vi "LD2018_ブロック崩し_当たり判定.vi"(0 "file path (dialog if empty)":path, 5 "Ball座標":T1, 7 "ブロックReferences":refnum<vi>[][](array[refnum]), 9 "ブロック配列in":bool[][](array[boolean]), 11 "方向in":i32, 12 "行":i32=10, 13 "列":i32=10) -> (6 "Hit?":bool, 10 "ブロック配列":bool[][](array[boolean]), 15 "方向out":i32)   [LabVIEW 2016]
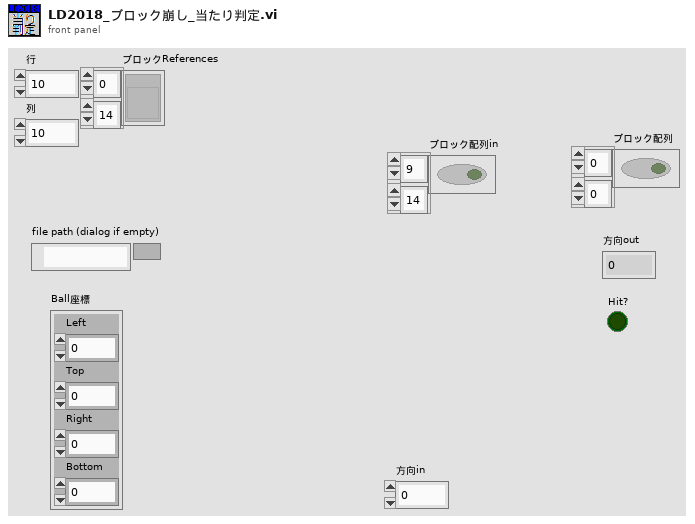
[diagram p1: front panel]
types:
  T1 = cluster{"Left":dbl, "Top":dbl, "Right":dbl, "Bottom":dbl}
  T2 = cluster{"Left":i16, "Top":i16, "Right":i16, "Bottom":i16}
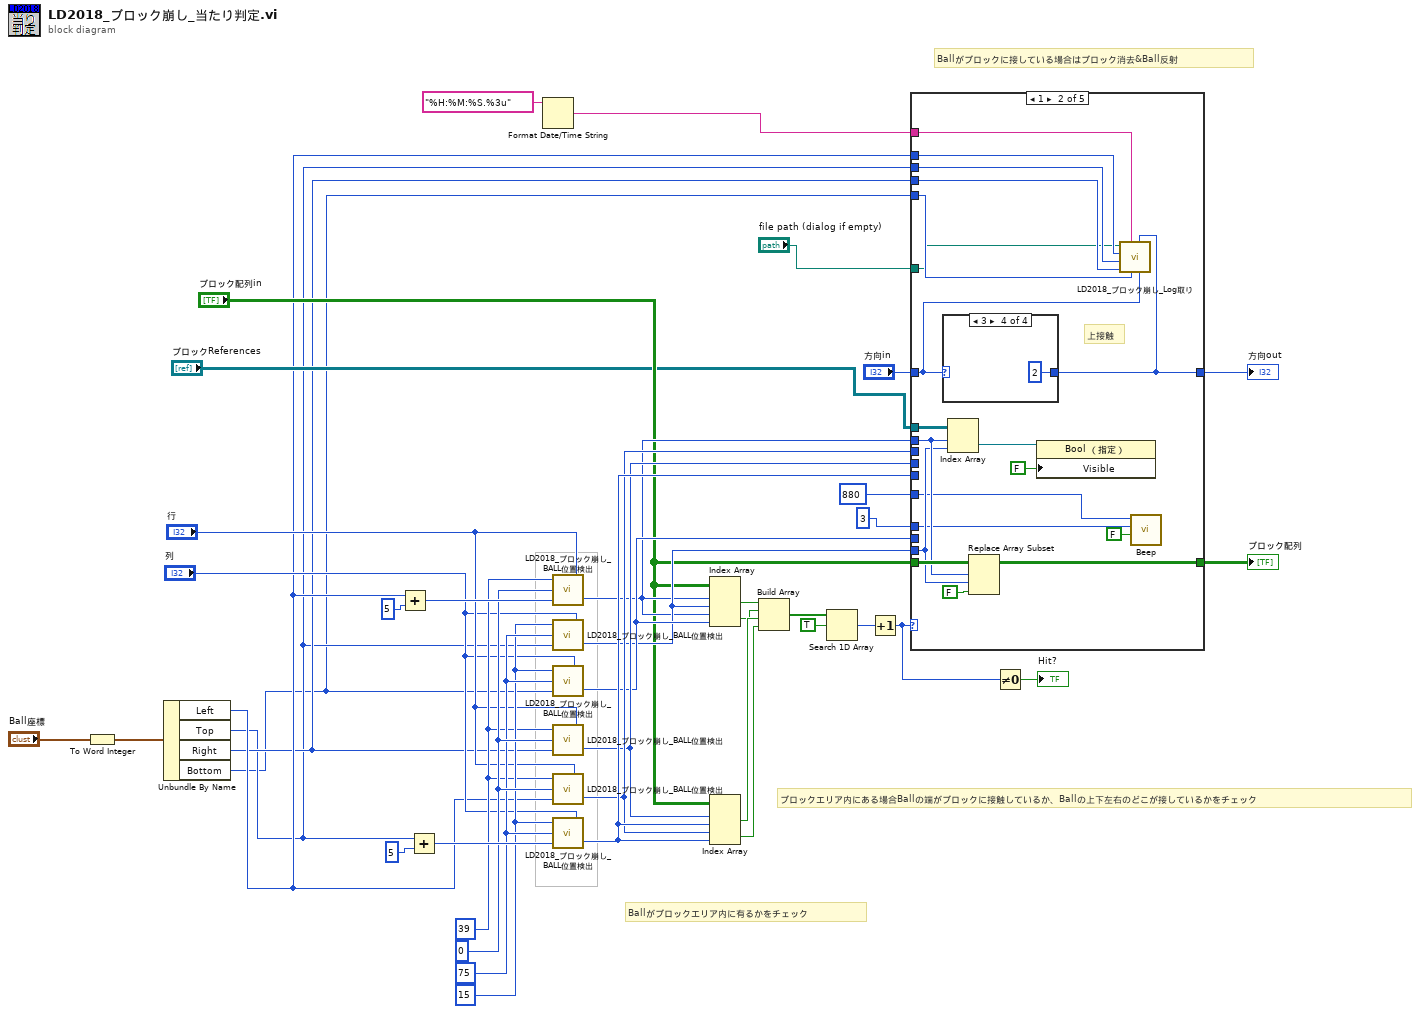
[diagram p0: block diagram]
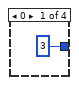
[diagram p3: hidden frame]
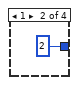
[diagram p4: hidden frame]
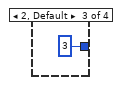
[diagram p5: hidden frame]
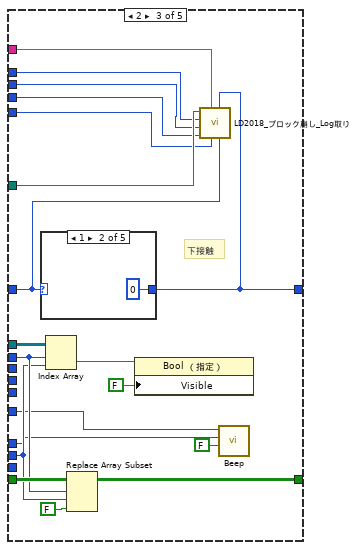
[diagram p6: hidden frame]
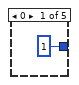
[diagram p7: hidden frame]
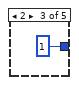
[diagram p8: hidden frame]
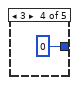
[diagram p9: hidden frame]
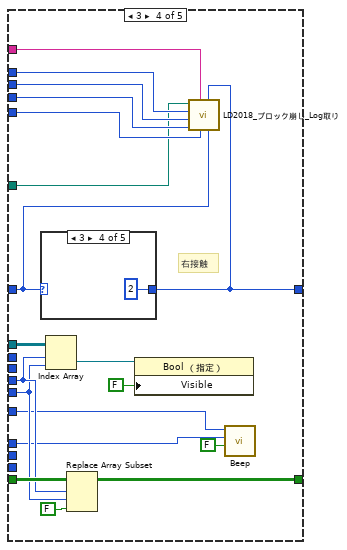
[diagram p11: hidden frame]
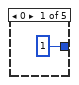
[diagram p12: hidden frame]
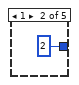
[diagram p13: hidden frame]
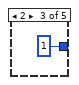
[diagram p14: hidden frame]
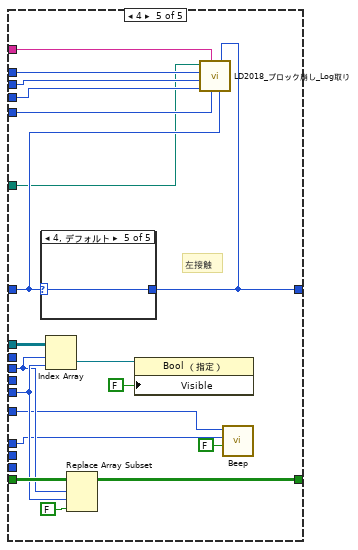
[diagram p16: hidden frame]
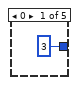
[diagram p17: hidden frame]
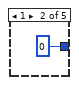
[diagram p18: hidden frame]
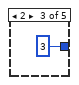
[diagram p19: hidden frame]
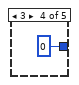
[diagram p20: hidden frame]
diagram:
  w19 = 75 ("オフセット")
  w20 = 0 ("オフセット")
  w17 = 39 ("幅/高さ")
  w18 = 15 ("幅/高さ")
  # "Ballがブロックに接している場合はブロック消去&Ball反射"
  # "ブロックエリア内にある場合Ballの端がブロックに接触しているか、Ballの上下左右のどこが接しているかをチェック"
  # "Ballがブロックエリア内に有るかをチェック"
  n1 = To Word Integer(number="Ball座標") -> (16bit integer=w3:T2)
  n2 = Unbundle By Name(w3) -> ("Left"=w7:i16, "Top"=w5:i16, "Right"=w6:i16, "Bottom"=w4:i16)
  n3 = Add(x=w7, y=i16 5) -> (x+y=w23:i16)
  n4 = Add(x=w5, y=i16 5) -> (x+y=w24:i16)
  n5 = Format Date/Time String(time format string (%c)="%H:%M:%S.%3u" ("時間形式文字列（%c）")) -> (date/time string=w11:string)  [unwired: 2 in]
  n6 = call "LD2018_ブロック崩し_BALL位置検出.vi"("行/列数"="行", "BALL座標"=w23, "オフセット"=w20, "幅/高さ"=w17) -> ("位置"=w33:i32)
  n7 = call "LD2018_ブロック崩し_BALL位置検出.vi"("行/列数"="列", "BALL座標"=w5, "オフセット"=w19, "幅/高さ"=w18) -> ("位置"=w34:i32)
  n8 = call "LD2018_ブロック崩し_BALL位置検出.vi"("行/列数"="列", "BALL座標"=w4, "オフセット"=w19, "幅/高さ"=w18) -> ("位置"=w35:i32)
  n9 = call "LD2018_ブロック崩し_BALL位置検出.vi"("行/列数"="行", "BALL座標"=w6, "オフセット"=w20, "幅/高さ"=w17) -> ("位置"=w36:i32)
  n10 = call "LD2018_ブロック崩し_BALL位置検出.vi"("行/列数"="行", "BALL座標"=w7, "オフセット"=w20, "幅/高さ"=w17) -> ("位置"=w37:i32)
  n11 = call "LD2018_ブロック崩し_BALL位置検出.vi"("行/列数"="列", "BALL座標"=w24, "オフセット"=w19, "幅/高さ"=w18) -> ("位置"=w38:i32)
  n12 = Index Array(array="ブロック配列in", index (row) #1=w33, index (col) #1=w34, index (row) #2=w33, index (col) #2=w35) -> (element #1=w26:bool, element #2=w27:bool)
  n13 = Index Array(array="ブロック配列in", index (row) #1=w36, index (col) #1=w38, index (row) #2=w37, index (col) #2=w38) -> (element #1=w28:bool, element #2=w29:bool)
  n14 = Build Array(w26, w27, w28, w29) -> (w30:bool[])
  n15 = Search 1D Array(1D array=w30, element=TRUE ("要素")) -> (index of element=w32:i32)  [unwired: 1 in]
  n16 = Increment(x=w32) -> (x+1=w10:i32)
  n17 = case shown="1" w10 {
    tunnel: w33 -> [_ w59 w82 _ _]
    tunnel: w34 -> [_ w58 _ _ _]
    tunnel: w35 -> [_ _ w78 _ _]
    tunnel: w36 -> [_ _ _ w103 _]
    tunnel: w37 -> [_ _ _ _ w126]
    tunnel: w38 -> [_ _ _ w102 w127]
    tunnel: "ブロック配列in" -> [w43 w62 w85 w109 w133]
    tunnel: "ブロックReferences" -> [_ w60 w83 w107 w131]
    tunnel: "方向in" -> [w42 w47 w72 w96 w120]
    tunnel: [w43 w55 w79 w104 w128] -> w40
    tunnel: [w42 w50 w71 w95 w118] -> w41
    tunnel: w7 -> [_ w54 w76 w100 w124]
    tunnel: w5 -> [_ w53 w75 w99 w123]
    tunnel: w6 -> [_ w52 w74 w98 w122]
    tunnel: w4 -> [_ w51 w73 w97 w121]
    tunnel: "file path (dialog if empty)" -> [_ w49 w77 w94 w119]
    tunnel: w11 -> [_ w48 w70 w101 w125]
    tunnel: u32 880 ("frequency (Hz)") -> [_ w45 w68 w92 w116]
    tunnel: u32 3 ("duration (msec)") -> [_ w44 w67 w91 w115]
    frame 0, Default {
    }
    frame 1 {
      # "上接触"
      n18 = case shown="3" w47 {
        tunnel: [3 ("y") 2 ("y") 3 ("y") 2 ("y")] -> w50
        frame 0 {
        }
        frame 1 {
        }
        frame 2, Default {
        }
        frame 3 {
        }
      }
      n19 = Index Array(array=w60, index (row)=w59, index (col)=w58) -> (element=w57:refnum<vi>)
      n20 = Replace Array Subset(array=w62, new element=FALSE ("新規要素/部分配列"), index (row)=w59, index (col)=w58) -> (w55:bool[][])
      n21 = property class="Bool （指定）"(reference=w57, "Visible"=FALSE ("表示")) -> ()  [unwired: 1 in, 2 out]
      n22 = call "LD2018_ブロック崩し_Log取り.vi"("方向 1"=w47, "方向 2"=w50, "BOTTOM"=w51, "time string"=w48, "R"=w52, "TOP"=w53, "L"=w54, "file path (dialog if empty)"=w49) -> ()  [unwired: 4 in]
      n23 = call <vilib>:"Beep.vi"("use system alert? (T)"=FALSE, "duration (msec)"=w44, "frequency (Hz)"=w45) -> ()  [unwired: 9 in]
    }
    frame 2 {
      # "下接触"
      n24 = case shown="1" w72 {
        selector: w72 -> [_ _ _ _ w90]
        tunnel: [1 ("y") 0 ("y") 1 ("y") 0 ("y") w90] -> w71
        frame 0 {
        }
        frame 1 {
        }
        frame 2 {
        }
        frame 3 {
        }
        frame 4, Default {
        }
      }
      n25 = Index Array(array=w83, index (row)=w82, index (col)=w78) -> (element=w81:refnum<vi>)
      n26 = Replace Array Subset(array=w85, new element=FALSE ("新規要素/部分配列"), index (row)=w82, index (col)=w78) -> (w79:bool[][])
      n27 = property class="Bool （指定）"(reference=w81, "Visible"=FALSE ("表示")) -> ()  [unwired: 1 in, 2 out]
      n28 = call "LD2018_ブロック崩し_Log取り.vi"("方向 1"=w72, "方向 2"=w71, "BOTTOM"=w73, "time string"=w70, "R"=w74, "TOP"=w75, "L"=w76, "file path (dialog if empty)"=w77) -> ()  [unwired: 4 in]
      n29 = call <vilib>:"Beep.vi"("use system alert? (T)"=FALSE, "duration (msec)"=w67, "frequency (Hz)"=w68) -> ()  [unwired: 9 in]
    }
    frame 3 {
      # "右接触"
      n30 = case shown="3" w96 {
        selector: w96 -> [_ _ _ _ w114]
        tunnel: [1 ("y") 2 ("y") 1 ("y") 2 ("y") w114] -> w95
        frame 0 {
        }
        frame 1 {
        }
        frame 2 {
        }
        frame 3 {
        }
        frame 4, Default {
        }
      }
      n31 = Index Array(array=w107, index (row)=w103, index (col)=w102) -> (element=w106:refnum<vi>)
      n32 = Replace Array Subset(array=w109, new element=FALSE ("新規要素/部分配列"), index (row)=w103, index (col)=w102) -> (w104:bool[][])
      n33 = property class="Bool （指定）"(reference=w106, "Visible"=FALSE ("表示")) -> ()  [unwired: 1 in, 2 out]
      n34 = call "LD2018_ブロック崩し_Log取り.vi"("方向 1"=w96, "方向 2"=w95, "BOTTOM"=w97, "time string"=w101, "R"=w98, "TOP"=w99, "L"=w100, "file path (dialog if empty)"=w94) -> ()  [unwired: 4 in]
      n35 = call <vilib>:"Beep.vi"("use system alert? (T)"=FALSE, "duration (msec)"=w91, "frequency (Hz)"=w92) -> ()  [unwired: 9 in]
    }
    frame 4 {
      # "左接触"
      n36 = case shown="4, デフォルト" w120 {
        selector: w120 -> [_ _ _ _ w138]
        tunnel: [3 ("y") 0 ("y") 3 ("y") 0 ("y") w138] -> w118
        frame 0 {
        }
        frame 1 {
        }
        frame 2 {
        }
        frame 3 {
        }
        frame 4, Default {
        }
      }
      n37 = Index Array(array=w131, index (row)=w126, index (col)=w127) -> (element=w130:refnum<vi>)
      n38 = Replace Array Subset(array=w133, new element=FALSE ("新規要素/部分配列"), index (row)=w126, index (col)=w127) -> (w128:bool[][])
      n39 = property class="Bool （指定）"(reference=w130, "Visible"=FALSE ("表示")) -> ()  [unwired: 1 in, 2 out]
      n40 = call "LD2018_ブロック崩し_Log取り.vi"("方向 1"=w120, "方向 2"=w118, "BOTTOM"=w121, "time string"=w125, "R"=w122, "TOP"=w123, "L"=w124, "file path (dialog if empty)"=w119) -> ()  [unwired: 4 in]
      n41 = call <vilib>:"Beep.vi"("use system alert? (T)"=FALSE, "duration (msec)"=w115, "frequency (Hz)"=w116) -> ()  [unwired: 9 in]
    }
  }
  "方向out" <- w41
  "ブロック配列" <- w40
  n42 = Not Equal To 0?(x=w10) -> (x != 0?=→"Hit?":bool)
